vi "Read Regression Line.vi"(6 "Maximum Time (10000 ms)":u32=10000, 7 "Data Source (0: Data Trace)":u16(ring) items=["Data Trace", "Memory Trace"], 8 "error in (no error)":errorcluster, 9 "Select Trace (1: 1)":u16(ring)=1 items=["1"=1, "2"=2, "3"=3, "4"=4], 10 "Measurement Type (3: Freq/Power)":u16(ring)=3 items=["Freq/Power"=3, "Transient"=5], 11 "VISA resource name":refnum<visa-resource-name>) -> (0 "error out":errorcluster, 1 "B":dbl format="%^#_9g", 2 "A":dbl format="%^#_9g", 3 "VISA resource name out":refnum<visa-resource-name>)   [LabVIEW 2011, in "Agilent E5052X.lvlib"]
doc: "Reads the \"A\" and \"B\" values of the regression line of either the memory or data trace. \n\n<b>Note: </b>\n\nThis VI applies to either Frequency/Power or Transient measurements."
uses:
  Agilent E5052X.lvlib
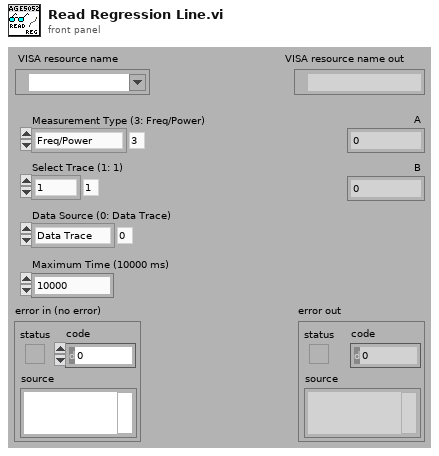
[diagram p1: front panel]
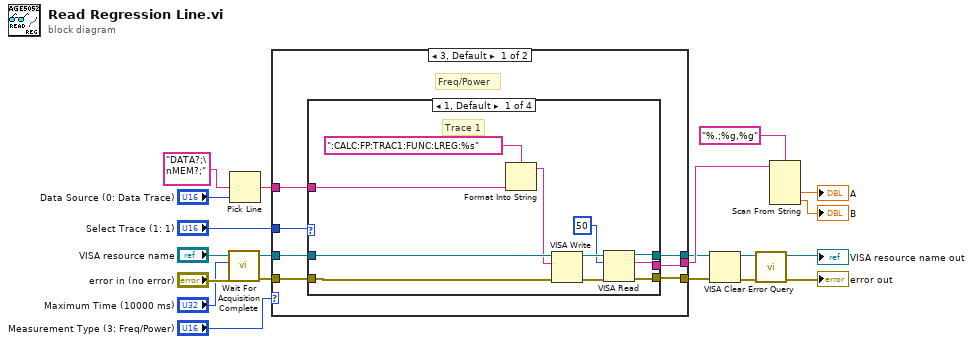
[diagram p0: block diagram]
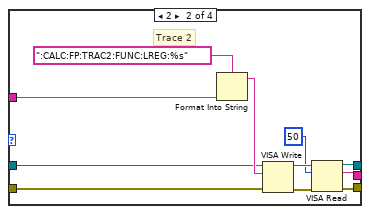
[diagram p2: hidden frame]
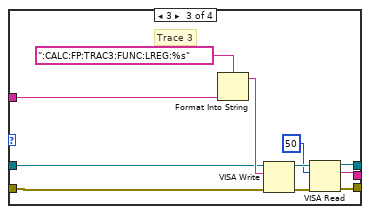
[diagram p3: hidden frame]
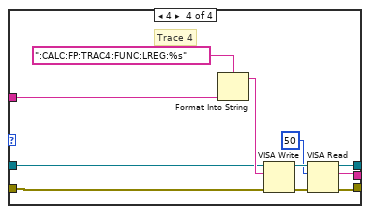
[diagram p4: hidden frame]
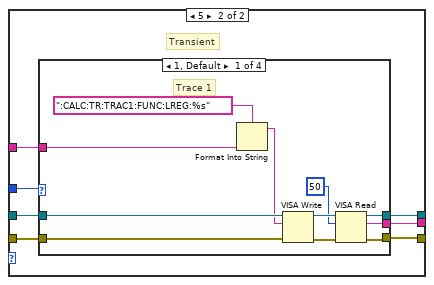
[diagram p5: hidden frame]
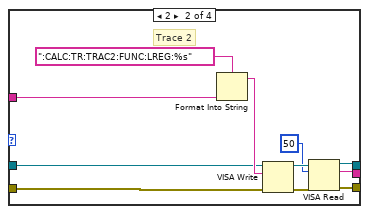
[diagram p6: hidden frame]
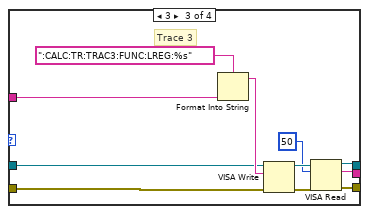
[diagram p7: hidden frame]
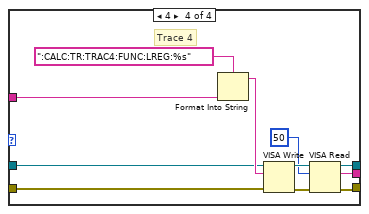
[diagram p8: hidden frame]
diagram:
  n1 = call "Wait For Acquisition Complete.vi"("error in (no error)"="error in (no error)", "Maximum Time (10000)"="Maximum Time (10000 ms)", "VISA resource name"="VISA resource name") -> ("error out"=w6:errorcluster, "VISA resource name out"=w7:refnum<visa-resource-name>)  [unwired: 7 in]
  n2 = Pick Line(multi-line string="DATA?;\nMEM?;", line index="Data Source (0: Data Trace)") -> (output string=w8:string)  [unwired: 1 in]
  n3 = case shown="3, Default" "Measurement Type (3: Freq/Power)" {
    tunnel: w6 -> [w24 w75]
    tunnel: w7 -> [w25 w76]
    tunnel: w8 -> [w26 w78]
    tunnel: "Select Trace (1: 1)" -> [w27 w77]
    tunnel: [w23 w74] -> w15
    tunnel: [w22 w73] -> w14
    tunnel: [w21 w72] -> w19
    frame 3, Default {
      # "Freq/Power"
      n4 = case shown="1, Default" w27 {
        tunnel: w26 -> [w38 w47 w58 w69]
        tunnel: w25 -> [w36 w46 w57 w68]
        tunnel: w24 -> [w35 w45 w56 w67]
        tunnel: [w30 w42 w52 w64] -> w23
        tunnel: [w29 w41 w55 w63] -> w22
        tunnel: [w28 w39 w50 w62] -> w21
        frame 1, Default {
          # "Trace 1"
          n5 = Format Into String(format string=":CALC:FP:TRAC1:FUNC:LREG:%s", w38) -> (resulting string=w34:string)  [unwired: 2 in, 1 out]
          n6 = VISA Write(VISA resource name=w36, write buffer=w34, error in (no error)=w35) -> (VISA resource name out=w33:refnum<visa-resource-name>, error out=w32:errorcluster)  [unwired: 1 out]
          n7 = VISA Read(VISA resource name=w33, byte count=u32 50, error in (no error)=w32) -> (VISA resource name out=w30:refnum<visa-resource-name>, read buffer=w28:string, error out=w29:errorcluster)  [unwired: 1 out]
        }
        frame 2 {
          # "Trace 2"
          n8 = Format Into String(format string=":CALC:FP:TRAC2:FUNC:LREG:%s", w47) -> (resulting string=w48:string)  [unwired: 2 in, 1 out]
          n9 = VISA Write(VISA resource name=w46, write buffer=w48, error in (no error)=w45) -> (VISA resource name out=w44:refnum<visa-resource-name>, error out=w43:errorcluster)  [unwired: 1 out]
          n10 = VISA Read(VISA resource name=w44, byte count=u32 50, error in (no error)=w43) -> (VISA resource name out=w42:refnum<visa-resource-name>, read buffer=w39:string, error out=w41:errorcluster)  [unwired: 1 out]
        }
        frame 3 {
          # "Trace 3"
          n11 = Format Into String(format string=":CALC:FP:TRAC3:FUNC:LREG:%s", w58) -> (resulting string=w59:string)  [unwired: 2 in, 1 out]
          n12 = VISA Write(VISA resource name=w57, write buffer=w59, error in (no error)=w56) -> (VISA resource name out=w54:refnum<visa-resource-name>, error out=w53:errorcluster)  [unwired: 1 out]
          n13 = VISA Read(VISA resource name=w54, byte count=u32 50, error in (no error)=w53) -> (VISA resource name out=w52:refnum<visa-resource-name>, read buffer=w50:string, error out=w55:errorcluster)  [unwired: 1 out]
        }
        frame 4 {
          # "Trace 4"
          n14 = Format Into String(format string=":CALC:FP:TRAC4:FUNC:LREG:%s", w69) -> (resulting string=w70:string)  [unwired: 2 in, 1 out]
          n15 = VISA Write(VISA resource name=w68, write buffer=w70, error in (no error)=w67) -> (VISA resource name out=w66:refnum<visa-resource-name>, error out=w65:errorcluster)  [unwired: 1 out]
          n16 = VISA Read(VISA resource name=w66, byte count=u32 50, error in (no error)=w65) -> (VISA resource name out=w64:refnum<visa-resource-name>, read buffer=w62:string, error out=w63:errorcluster)  [unwired: 1 out]
        }
      }
    }
    frame 5 {
      # "Transient"
      n17 = case shown="1, Default" w77 {
        tunnel: w78 -> [w89 w98 w109 w120]
        tunnel: w76 -> [w87 w97 w108 w119]
        tunnel: w75 -> [w86 w96 w107 w118]
        tunnel: [w81 w92 w103 w116] -> w74
        tunnel: [w80 w95 w106 w115] -> w73
        tunnel: [w79 w91 w101 w117] -> w72
        frame 1, Default {
          # "Trace 1"
          n18 = Format Into String(format string=":CALC:TR:TRAC1:FUNC:LREG:%s", w89) -> (resulting string=w85:string)  [unwired: 2 in, 1 out]
          n19 = VISA Write(VISA resource name=w87, write buffer=w85, error in (no error)=w86) -> (VISA resource name out=w83:refnum<visa-resource-name>, error out=w84:errorcluster)  [unwired: 1 out]
          n20 = VISA Read(VISA resource name=w83, byte count=u32 50, error in (no error)=w84) -> (VISA resource name out=w81:refnum<visa-resource-name>, read buffer=w79:string, error out=w80:errorcluster)  [unwired: 1 out]
        }
        frame 2 {
          # "Trace 2"
          n21 = Format Into String(format string=":CALC:TR:TRAC2:FUNC:LREG:%s", w98) -> (resulting string=w99:string)  [unwired: 2 in, 1 out]
          n22 = VISA Write(VISA resource name=w97, write buffer=w99, error in (no error)=w96) -> (VISA resource name out=w94:refnum<visa-resource-name>, error out=w93:errorcluster)  [unwired: 1 out]
          n23 = VISA Read(VISA resource name=w94, byte count=u32 50, error in (no error)=w93) -> (VISA resource name out=w92:refnum<visa-resource-name>, read buffer=w91:string, error out=w95:errorcluster)  [unwired: 1 out]
        }
        frame 3 {
          # "Trace 3"
          n24 = Format Into String(format string=":CALC:TR:TRAC3:FUNC:LREG:%s", w109) -> (resulting string=w110:string)  [unwired: 2 in, 1 out]
          n25 = VISA Write(VISA resource name=w108, write buffer=w110, error in (no error)=w107) -> (VISA resource name out=w105:refnum<visa-resource-name>, error out=w104:errorcluster)  [unwired: 1 out]
          n26 = VISA Read(VISA resource name=w105, byte count=u32 50, error in (no error)=w104) -> (VISA resource name out=w103:refnum<visa-resource-name>, read buffer=w101:string, error out=w106:errorcluster)  [unwired: 1 out]
        }
        frame 4 {
          # "Trace 4"
          n27 = Format Into String(format string=":CALC:TR:TRAC4:FUNC:LREG:%s", w120) -> (resulting string=w121:string)  [unwired: 2 in, 1 out]
          n28 = VISA Write(VISA resource name=w119, write buffer=w121, error in (no error)=w118) -> (VISA resource name out=w113:refnum<visa-resource-name>, error out=w114:errorcluster)  [unwired: 1 out]
          n29 = VISA Read(VISA resource name=w113, byte count=u32 50, error in (no error)=w114) -> (VISA resource name out=w116:refnum<visa-resource-name>, read buffer=w117:string, error out=w115:errorcluster)  [unwired: 1 out]
        }
      }
    }
  }
  n30 = VISA Clear(VISA resource name=w15, error in (no error)=w14) -> (VISA resource name out=w2:refnum<visa-resource-name>, error out=w1:errorcluster)
  n31 = call "Error Query.vi"("error in (no error)"=w1, "VISA resource name"=w2) -> ("error out"=→"error out":errorcluster, "VISA resource name out"=→"VISA resource name out":refnum<visa-resource-name>)  [unwired: 6 in, 2 out]
  n32 = Scan From String(format string="%.;%g,%g", input string=w19) -> (output 1=→"A":dbl, output 2=→"B":dbl)  [unwired: 4 in, 3 out]
